vi "Create Protected Pointer Error.vi"(7 "source vi name":string, 11 "error":T1) -> (1 "new offset":i32, 3 "error out":errorcluster)   [LabVIEW 2017, in "Memory Manager.lvlib" / "Protected Pointer.lvclass"]
uses:
  Protected Pointer.lvclass
  Errors.ctl
  Constants/Library Name.vi
  VIs/VIs for Poly/Create Error Cluster (512B).vi
  Memory Manager.lvlib
  Deterministic Error Builder.lvlib
  <vilib>/NI/Static Error Handling/Static Error Handling.lvlib
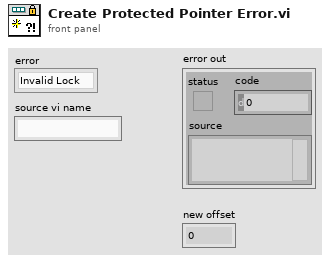
[diagram p1: front panel]
types:
  T1 = typedef "Memory Manager.lvlib/Protected Pointer.lvclass/Errors.ctl" = enum16{"Invalid Lock"}
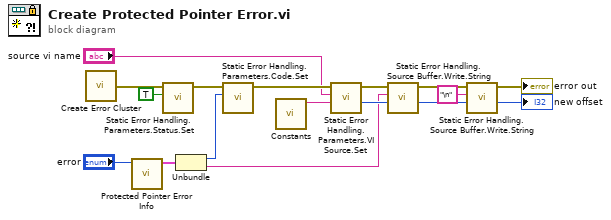
[diagram p0: block diagram]
diagram:
  n1 = call-poly "Create Error Cluster.vi"() -> ("error out"=w5:errorcluster)  [unwired: 1 in]
  n2 = call "Protected Pointer Error Info.vi"("error"="error") -> ("error info"=w4:cluster{"code":i32, "description":string})  [unwired: 10 in]
  n3 = call <vilib>:"Static Error Handling.Parameters.Status.Set.vi"("status (T)"=TRUE, "error in"=w5) -> ("error out"=w15:errorcluster)  [unwired: 9 in]
  n4 = Unbundle(w4) -> ("code"=w12:i32, "description"=w9:string)
  n5 = call <vilib>:"Static Error Handling.Parameters.Code.Set.vi"("code"=w12, "error in"=w15) -> ("error out"=w16:errorcluster)  [unwired: 9 in]
  n6 = call-poly "Constants.vi"() -> ("library name"=w17:string)  [unwired: 11 in]
  n7 = call <vilib>:"Static Error Handling.Parameters.VI Source.Set.vi"("library name (\"\")"=w17, "vi name"="source vi name", "error in"=w16) -> ("new offset"=w10:i32, "error out"=w11:errorcluster)  [unwired: 7 in]
  n8 = call <vilib>:"Static Error Handling.Source Buffer.Write.String.vi"("offset"=w10, "string"=w9, "error in"=w11) -> ("new offset"=w7:i32, "error out"=w8:errorcluster)  [unwired: 7 in]
  n9 = call <vilib>:"Static Error Handling.Source Buffer.Write.String.vi"("offset"=w7, "string"="\n", "error in"=w8) -> ("new offset"=→"new offset":i32, "error out"=→"error out":errorcluster)  [unwired: 7 in]
